vi "test_Add Static Scalar Input Channels.vi"(8 "error in (no error)":errorcluster, 11 "TestCase in":refnum<class "FPGA Addon Adding Channel Items Unit Tests.lvclass">) -> (0 "error out":errorcluster, 3 "TestCase out":refnum<class "FPGA Addon Adding Channel Items Unit Tests.lvclass">)   [LabVIEW 2020, in "FPGA Addon Adding Channel Items Unit Tests.lvclass"]
uses:
  FPGA Addon Adding Channel Items Unit Tests.lvclass
  <vilib>/NI VeriStand/Custom Device API/Custom Device Channel.ctl
  <vilib>/NI VeriStand/Custom Device API/Custom Device Channel Type.ctl
  Addon/Addon System Explorer/Types/Channel Type.ctl
  Addon/Addon System Explorer/Types/SE UI Cluster.ctl
  <vilib>/NI VeriStand/Custom Device API/Custom Device Item Ref.ctl
  FPGA Addon Adding Channel Items Unit Tests.lvclass/FPGA Addon Adding Channel Items Unit Tests.ctl
  Addon/Addon Shared/SubVIs/Constants.vi
  <vilib>/NI VeriStand/Custom Device Tools/Custom Device Utility Library/NI VeriStand - Search for Item by GUID.vi
  <vilib>/NI/NI VeriStand Advanced SysDef API/_SubVIs/SysDef.Search.GUIDs.vi
  <vilib>/addons/_JKI Toolkits/VI Tester/TestCase.llb/TestCase.lvclass
  Addon/Addon System Explorer/FPGA Addon System Explorer.lvlib
  <vilib>/NI VeriStand/Custom Device Tools/Custom Device Utility Library/Custom Device Utility Library.lvlib
  Addon/Addon Shared/FPGA Addon Shared.lvlib
  <vilib>/NI/NI VeriStand Advanced SysDef API/SysDef API/Advanced System Definition.lvlib
  <vilib>/NI VeriStand/Custom Device API/Custom Device API.lvlib
  C:/Program Files (x86)/National Instruments/LabVIEW 2020/vi.lib/addons/_JKI Toolkits/VI Tester/TestCase.llb/TestCase.lvclass
panel:
  out "GUIDs":string[](array[string])
  out "Channels":T1[](array[typedef])
  in  "remove":bool
  in  "add":bool
  out "Names":string[](array[string])
  in  "Available Registers":i32[](listbox)
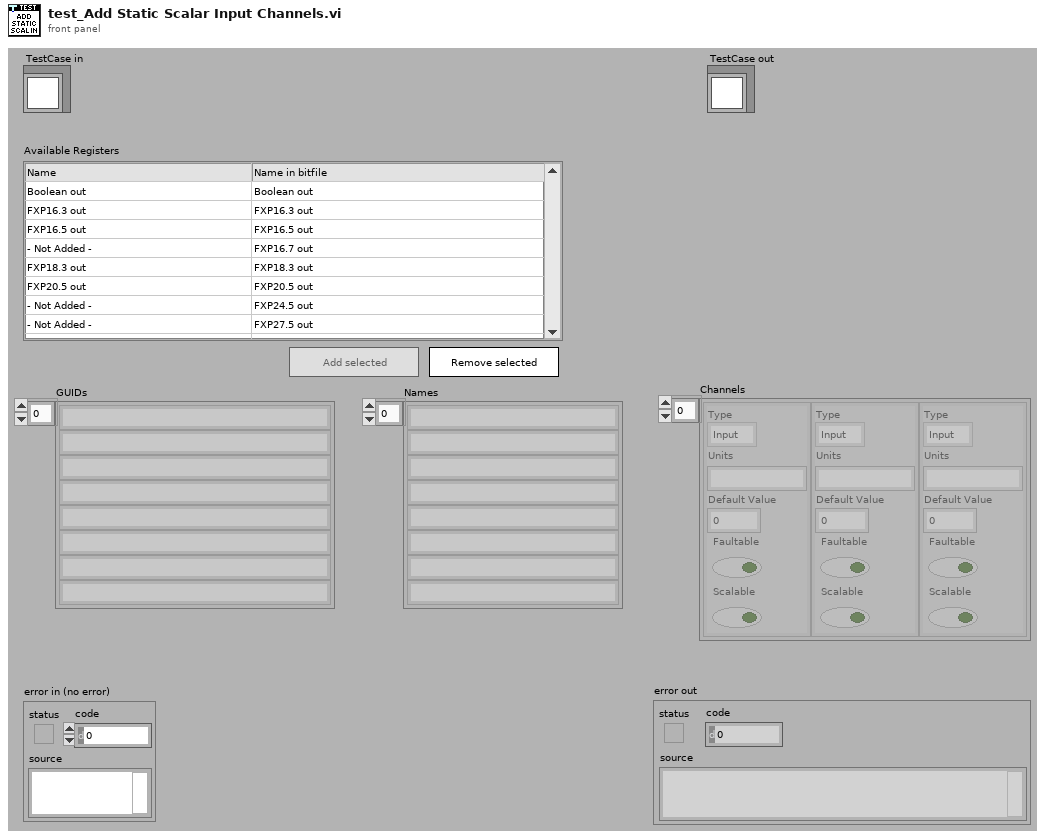
[diagram p1: front panel]
types:
  T1 = typedef "Custom Device API.lvlib/Custom Device Channel.ctl" = cluster{"Type":T2, "Units":string, "Default Value":dbl, "Faultable":bool, "Scalable":bool}
  T2 = typedef "Custom Device API.lvlib/Custom Device Channel Type.ctl" = enum16{"Input", "Output"}
  T3 = typedef "FPGA Addon System Explorer.lvlib/SE UI Cluster.ctl" = cluster{"Node Ptr":T4, "Add":refnum<vi>, "Remove":refnum<vi>, "Registers ListBox":refnum<vi>}
  T4 = typedef "Custom Device API.lvlib/Custom Device Item Ref.ctl" = u64
  T5 = typedef "FPGA Addon System Explorer.lvlib/Channel Type.ctl" = enum16{"Write Channel", "Read Channel", "Write Waveform", "Read Waveform"}
  T6 = typedef "Advanced System Definition.lvlib/TreeItem.Info.ctl" = cluster{"Name":string, "Description":string, "GUID":string, "Is Channel":bool, "Channel":T1, "Is Waveform":bool, "Waveform":T7}
  T7 = typedef "Custom Device API.lvlib/Custom Device Waveform.ctl" = cluster{"Data Type":T8, "Units":string}
  T8 = typedef "Custom Device API.lvlib/Custom Device Waveform DataType.ctl" = enum16{"Double", "Complex Double"}
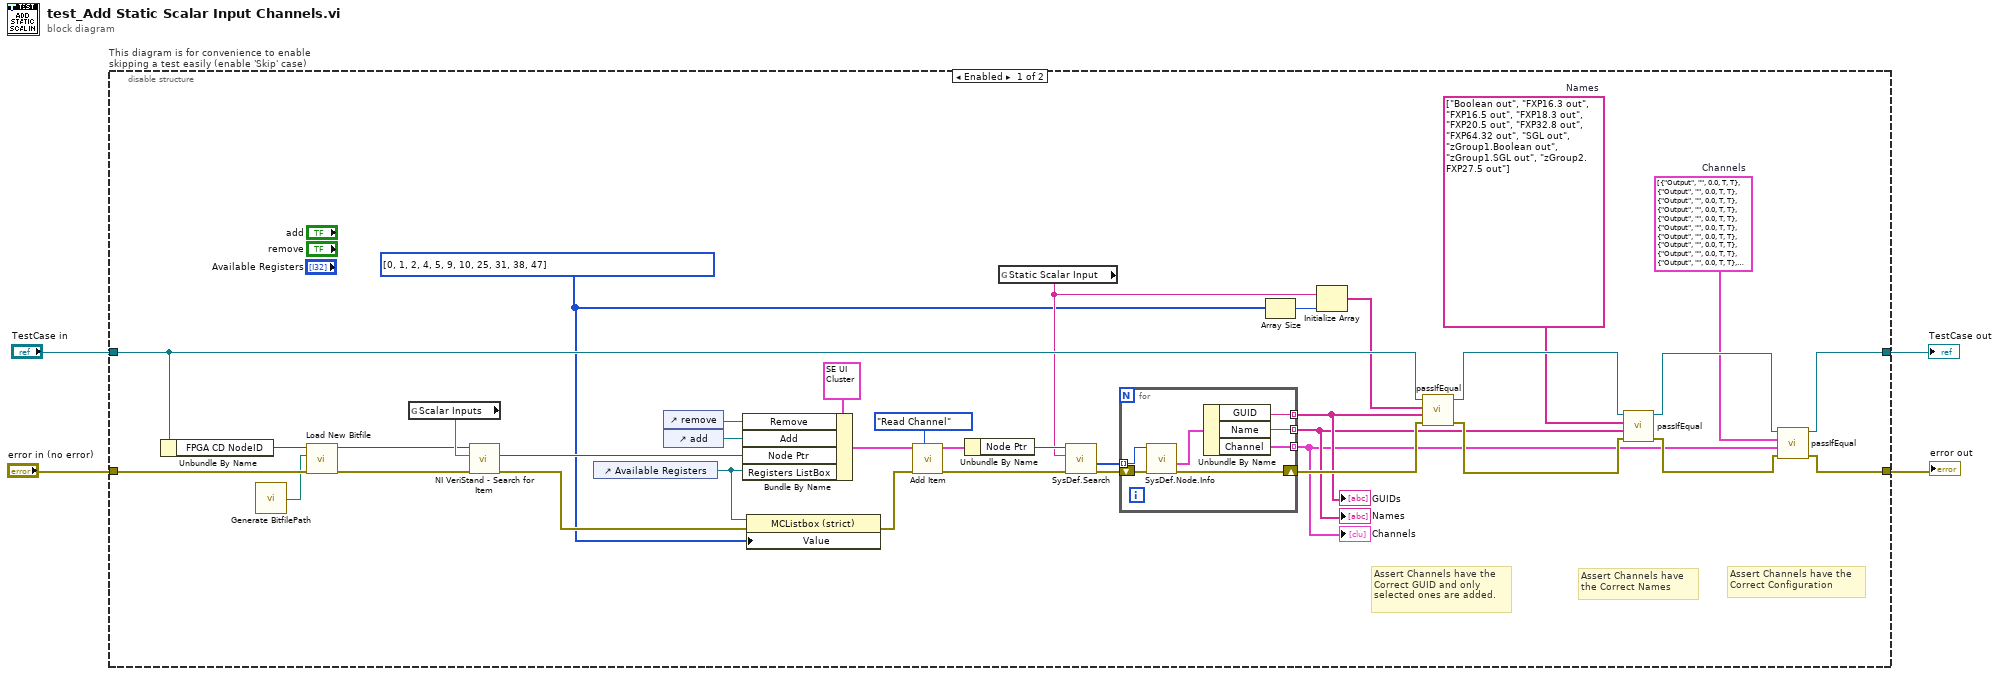
[diagram p0: block diagram]
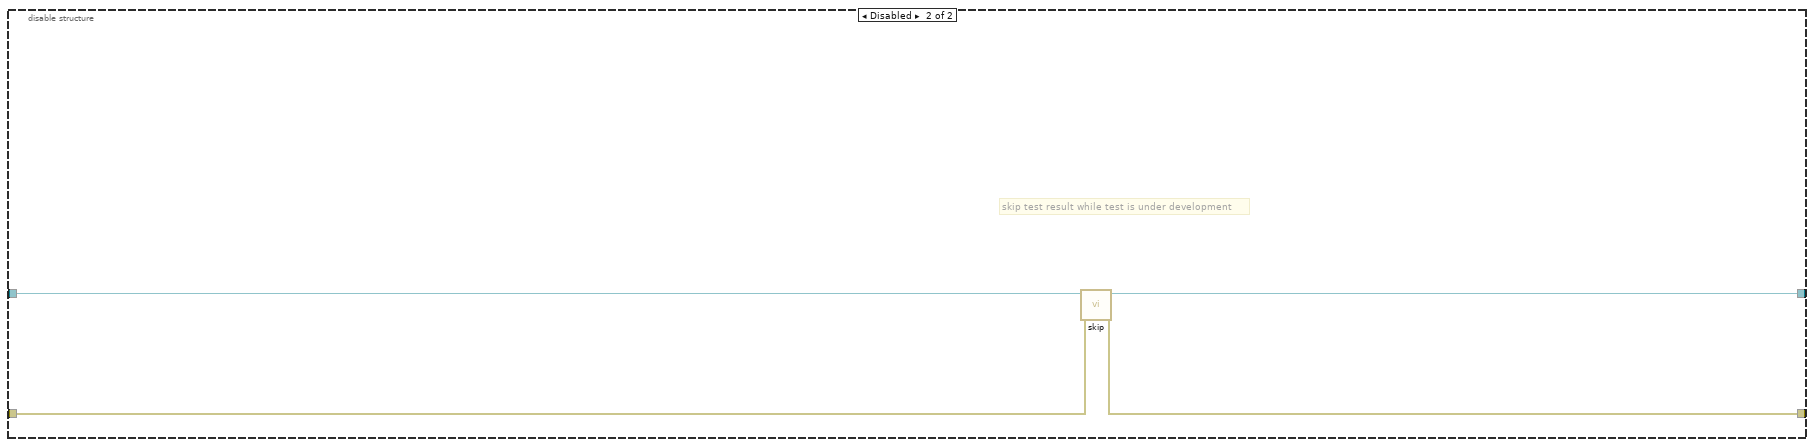
[diagram p2: hidden frame]
diagram:
  n1 = disable-structure "This diagram is for convenience to enable skipping a test easily (enable 'Skip' case)" shown="Enabled" {
    disable-tunnel: "TestCase in" -> [w33 w52]
    disable-tunnel: [w29 w50] -> w1
    disable-tunnel: [w26 w51] -> w3
    disable-tunnel: "error in (no error)" -> [w22 w49]
    frame Enabled {
      w24 = T1[] [{"Type"=enum."Output", "Units"="", "Default Value"=0.0, "Faultable"=TRUE, "Scalable"=TRUE}, {"Type"=enum."Output", "Units"="", "Default Value"=0.0, "Faultable"=TRUE, "Scalable"=TRUE}, {"Type"=enum."Output", "Units"="", "Default Value"=0.0, "Faultable"=TRUE, "Scalable"=TRUE}, {"Type"=enum."Output", "Units"="", "Default Value"=0.0, "Faultable"=TRUE, "Scalable"=TRUE}, {"Type"=enum."Output", "Units"="", "Default Value"=0.0, "Faultable"=TRUE, "Scalable"=TRUE}, {"Type"=enum."Output", "Units"="", "Default Value"=0.0, "Faultable"=TRUE, "Scalable"=TRUE}, {"Type"=enum."Output", "Units"="", "Default Value"=0.0, "Faultable"=TRUE, "Scalable"=TRUE}, {"Type"=enum."Output", "Units"="", "Default Value"=0.0, "Faultable"=TRUE, "Scalable"=TRUE}, {"Type"=enum."Output", "Units"="", "Default Value"=0.0, "Faultable"=TRUE, "Scalable"=TRUE}, {"Type"=enum."Output", "Units"="", "Default Value"=0.0, "Faultable"=TRUE, "Scalable"=TRUE}, {"Type"=enum."Output", "Units"="", "Default Value"=0.0, "Faultable"=TRUE, "Scalable"=TRUE}]  # Channels
      w30 = string[] ["Boolean out", "FXP16.3 out", "FXP16.5 out", "FXP18.3 out", "FXP20.5 out", "FXP32.8 out", "FXP64.32 out", "SGL out", "zGroup1.Boolean out", "zGroup1.SGL out", "zGroup2.FXP27.5 out"]  # Names
      w6 = i32[] [0, 1, 2, 4, 5, 9, 10, 25, 31, 38, 47] ("selected")
      # "Assert Channels have the Correct Configuration"
      # "Assert Channels have the Correct Names"
      # "Assert Channels have the Correct GUID and only selected ones are added."
      n2 = Unbundle By Name(w33) -> ("FPGA CD NodeID"=w21:u64)
      n3 = call "Generate BitfilePath.vi"() -> ("Bitfile path"=w20:path)
      n4 = call "Load New Bitfile.vi"("error in (no error)"=w22, "NewVal"=w20, "Item Ref in"=w21) -> ("error out"=w23:errorcluster, "Section Ref out"=w19:T4)  [unwired: 7 in]
      n5 = global read "Constants.vi" "Scalar Inputs"() -> (w40:string)
      n6 = call-poly <vilib>:"NI VeriStand - Search for Item.vi"("error in"=w23, "Item GUID"=w40, "Section Ref in"=w19) -> ("error out"=w7:errorcluster, "Item Ref"=w12:T4)  [unwired: 5 in, 2 out]
      n7 = control-ref of="Available Registers"() -> (w8:refnum<vi>)
      n8 = control-ref of="remove"() -> (w10:refnum<vi>)
      n9 = control-ref of="add"() -> (w9:refnum<vi>)
      n10 = Bundle By Name(cluster=T3 {"Node Ptr"=18446744073709551615, "Add"=refnum, "Remove"=refnum, "Registers ListBox"=refnum} ("SE UI cluster in"), "Remove"=w10, "Add"=w9, "Node Ptr"=w12, "Registers ListBox"=w8) -> (w11:T3)
      n11 = property class="MCListbox (strict)"(reference=w8, error in=w7, "Value"=w6) -> (error out=w5:errorcluster)  [unwired: 1 out]
      n12 = call "Add Item.vi"("Action"=Channel_Type."Read Channel", "error in (no error)"=w5, "SE UI cluster in"=w11) -> ("error out"=w18:errorcluster, "SE UI cluster out"=w17:T3)  [unwired: 7 in]
      n13 = Unbundle By Name(w17) -> ("Node Ptr"=w38:T4)
      n14 = global read "Constants.vi" "Static Scalar Input"() -> (w15:string)
      n15 = call-poly <vilib>:"SysDef.Search.vi"("error in (no error)"=w18, "GUID"=w15, "nodeID"=w38) -> ("error out"=w39:errorcluster, "Values Out"=w37:u64[])  [unwired: 5 in, 2 out]
      n16 = for {
        tunnel: w37 -> [w44] mode=indexing
        tunnel: [w42] -> w31 mode=indexing
        tunnel: [w45] -> w25 mode=indexing
        tunnel: [w43] -> w34 mode=indexing
        shift-right: [w47] -> w35
        shift-left: w39 -> [w48]
        n17 = call <vilib>:"SysDef.Node.Info.vi"("error in (no error)"=w48, "nodeID"=w44) -> ("error out"=w47:errorcluster, "Item Info"=w46:T6)  [unwired: 6 in, 2 out]
        n18 = Unbundle By Name(w46) -> ("GUID"=w43:string, "Name"=w42:string, "Channel"=w45:T1)
      }
      "Names" <- w31
      "Channels" <- w25
      "GUIDs" <- w34
      n19 = Array Size(array=w6) -> (size(s)=w14:i32)
      n20 = Initialize Array(w15, w14) -> (w16:string[])
      n21 = call-dynamic "passIfEqual.vi"("error in (no error)"=w35, "y"=w34, "x"=w16, "TestCase in"=w33) -> ("error out"=w36:errorcluster, "TestCase out"=w32:refnum<class "FPGA Addon Adding Channel Items Unit Tests.lvclass">)  [unwired: 6 in]
      n22 = call-dynamic "passIfEqual.vi"("error in (no error)"=w36, "y"=w31, "x"=w30, "TestCase in"=w32) -> ("error out"=w27:errorcluster, "TestCase out"=w28:refnum<class "FPGA Addon Adding Channel Items Unit Tests.lvclass">)  [unwired: 6 in]
      n23 = call-dynamic "passIfEqual.vi"("error in (no error)"=w27, "y"=w25, "x"=w24, "TestCase in"=w28) -> ("error out"=w26:errorcluster, "TestCase out"=w29:refnum<class "FPGA Addon Adding Channel Items Unit Tests.lvclass">)  [unwired: 6 in]
    }
    frame Disabled {
      # "skip test result while test is under development"
      n24 = call <vilib>:"skip.vi"("error in (no error)"=w49, "TestCase in"=w52) -> ("error out"=w51:errorcluster, "TestCase out"=w50:refnum<class "FPGA Addon Adding Channel Items Unit Tests.lvclass">)  [unwired: 8 in]
    }
  }
  "error out" <- w3
  "TestCase out" <- w1
